vi "rt_loop_message_handling.vi"(8 "error in (no error)":errorcluster caption="错误输入（无错误）", 11 "Message Queues":T1 caption="消息队列") -> (0 "error out":errorcluster caption="错误输出")   [LabVIEW 2015]
uses:
  support_vis/message_queue/all_rt_message_queues.ctl
  support_vis/message_queue/message_cluster.ctl
  globals/global_monitoring_variables.vi
  globals/global_device_tree_items.vi
  globals/global_configuration_options.vi
  globals/global_all_rt_loop_stop.vi
  globals/global_rt_stream_connections.vi
  support_vis/message_queue/message_queue.lvlib
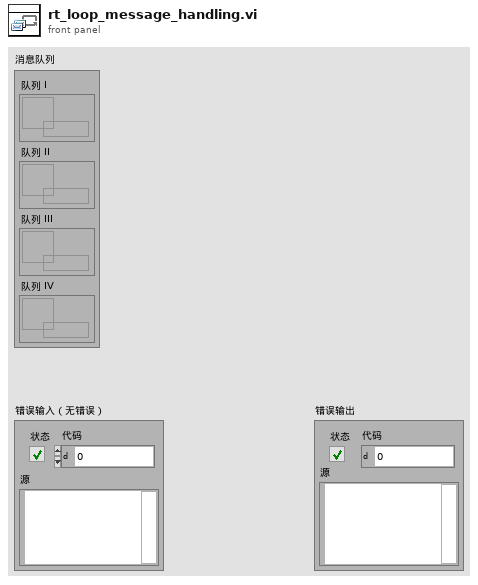
[diagram p1: front panel]
types:
  T1 = typedef "message_queue.lvlib/all_rt_message_queues.ctl" = cluster{"Queue I":refnum<queue>, "Queue II":refnum<queue>, "Queue III":refnum<queue>, "Queue IV":refnum<queue>}
  T2 = cluster{"Left Cell String":string, "Child Text":string[], "Child Tag":string, "Item Indent":i32, "Child Only?":bool, "Glyph Index":i32}[]
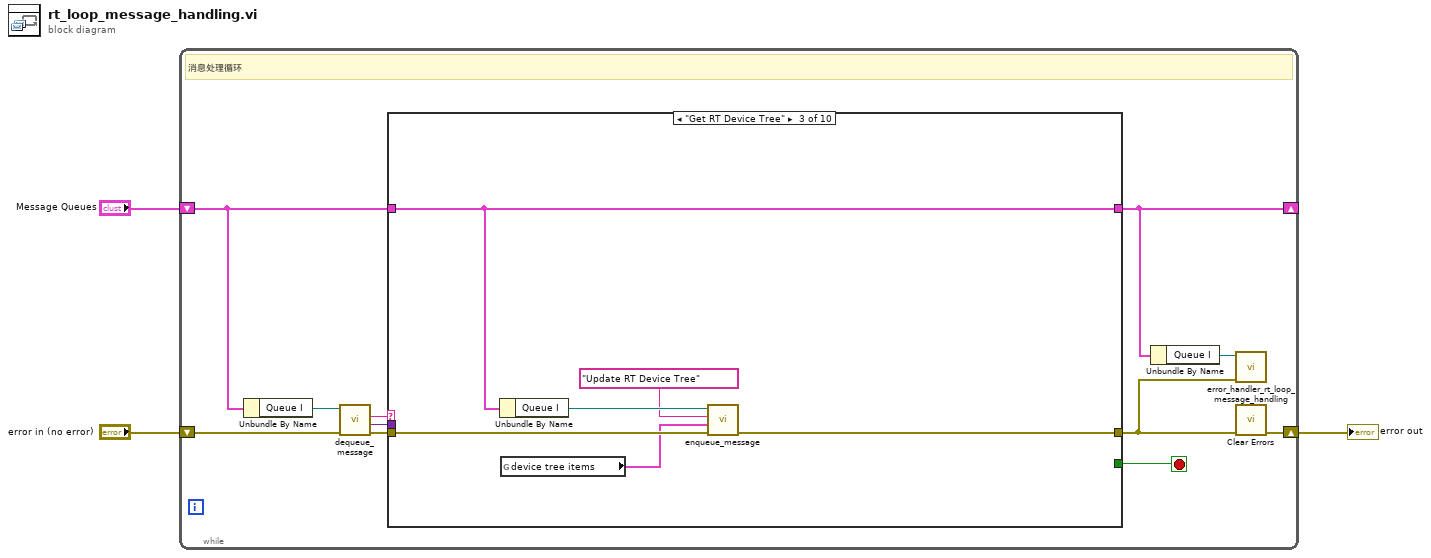
[diagram p0: block diagram]
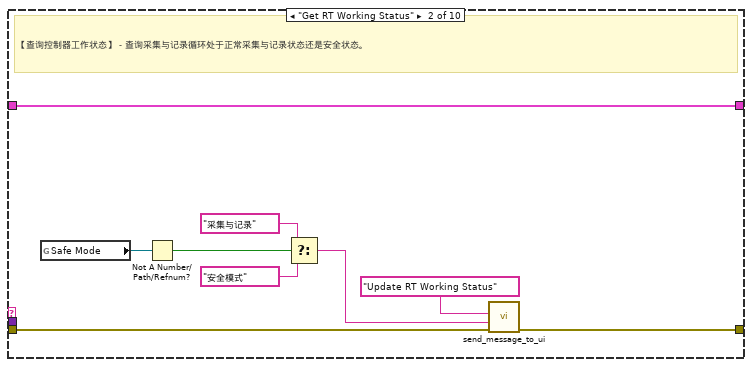
[diagram p3: hidden frame]
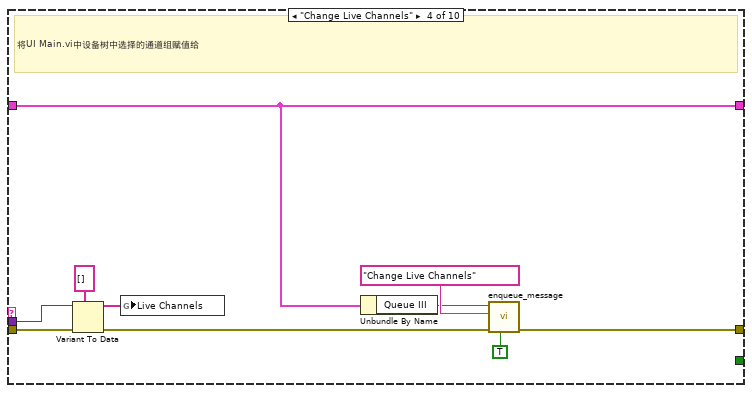
[diagram p4: hidden frame]
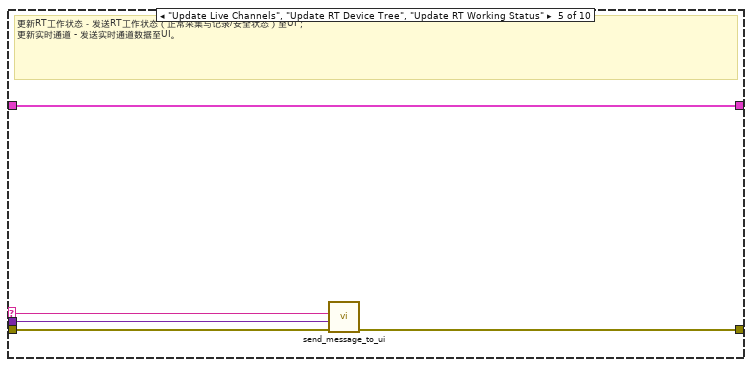
[diagram p5: hidden frame]
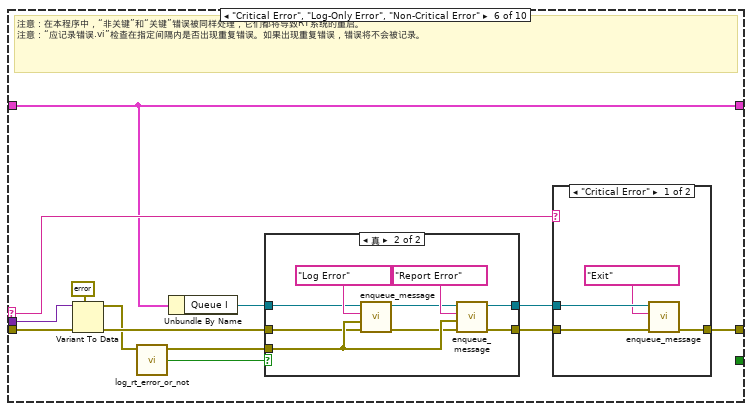
[diagram p6: hidden frame]
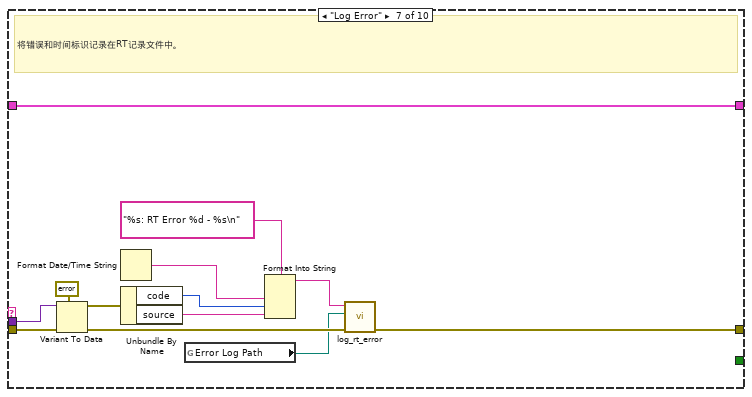
[diagram p9: hidden frame]
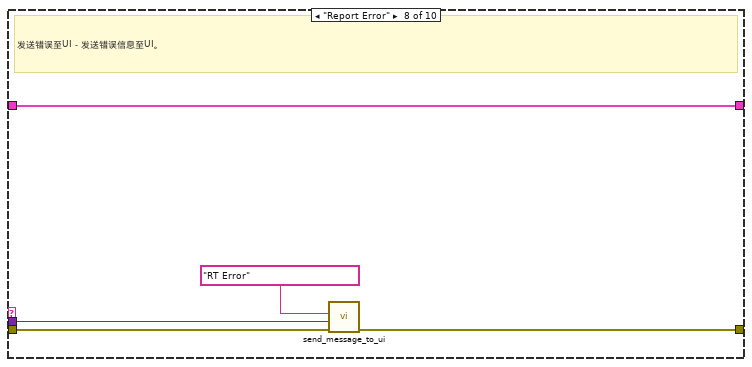
[diagram p10: hidden frame]
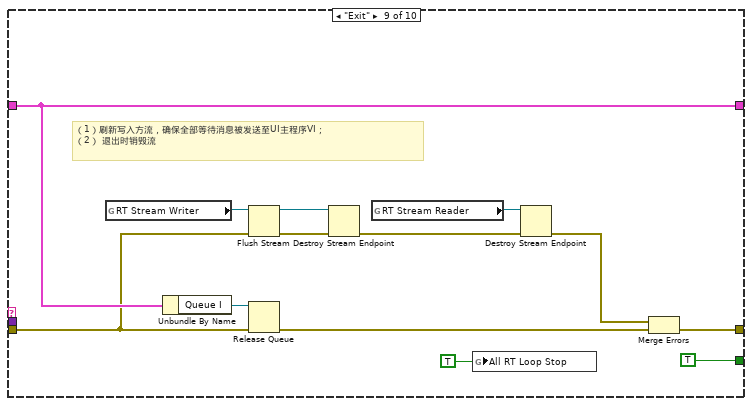
[diagram p11: hidden frame]
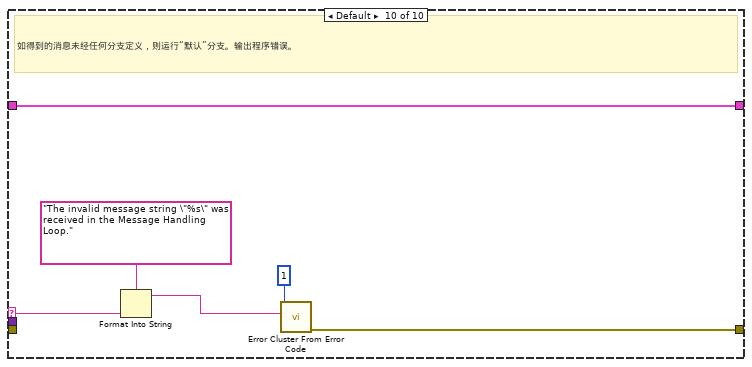
[diagram p12: hidden frame]
diagram:
  n1 = while {
    shift-right: [w9] -> w2
    shift-left: "error in (no error)" -> [w13]
    shift-right: [w6] -> _
    shift-left: "Message Queues" -> [w7]
    stop <- w14 stop-if-true
    # "消息处理循环"
    n2 = Unbundle By Name(w7) -> ("Queue I"=w5:refnum<queue>)
    n3 = call "dequeue_message.vi"("error in (no error)"=w13, "Message Queue"=w5) -> ("error out"=w12:errorcluster, "Message Data"=w10:variant, "Message"=w11:string)  [unwired: 6 in, 1 out]
    n4 = case "Message Cases" shown="\"Get RT Device Tree\"" w11 {
      selector: w11 -> [_ _ _ _ w42 w54 _ _ _ w111]
      tunnel: w12 -> [w16 w20 w27 w41 w46 w56 w88 w93 w96 _]
      tunnel: [w16 w19 w31 w36 w45 w59 w79 w92 w95 w109] -> w8
      tunnel: [_ _ _ _ _ _ _ _ TRUE _] -> w14
      tunnel: w10 -> [_ _ _ w39 w44 w49 w87 w91 _ _]
      tunnel: w7 -> [w15 w25 w30 w33 w43 w48 w76 w90 w99 w107]
      tunnel: [w15 w25 w30 w33 w43 w48 w76 w90 w99 w107] -> w6
      frame "Initialize" {
      }
      frame "Get RT Working Status" {
        # "【查询控制器工作状态】－查询采集与记录循环处于正常采集与记录状态还是安全状态。"
        n5 = global read "global_monitoring_variables.vi" "Safe Mode"() -> (w24:refnum<k4>)
        n6 = Not A Number/Path/Refnum?(number/path/refnum=w24) -> (NaN/Path/Refnum?=w23:bool)
        n7 = Select(t="采集与记录", s=w23, f="安全模式") -> (s? t:f=w18:string)
        n8 = call "send_message_to_ui.vi"("error in (no error)"=w20, "Message Data"=w18, "Message"="Update RT Working Status") -> ("error out"=w19:errorcluster)  [unwired: 8 in]
      }
      frame "Get RT Device Tree" {
        n9 = Unbundle By Name(w30) -> ("Queue I"=w29:refnum<queue>)
        n10 = global read "global_device_tree_items.vi" "device tree items"() -> (w26:T2)
        n11 = call "enqueue_message.vi"("error in (no error)"=w27, "Message Data"=w26, "Message"="Update RT Device Tree", "Message Queue"=w29) -> ("error out"=w31:errorcluster)  [unwired: 6 in, 1 out]
      }
      frame "Change Live Channels" {
        # "将UI Main.vi中设备树中选择的通道组赋值给"
        n12 = Variant To Data(error in=w41, type=string[] [] ("Displaying Channels"), Variant=w39) -> (data=w37:string[], error out=w40:errorcluster)
        n13 = global write "global_monitoring_variables.vi" "Live Channels"(w37) -> ()
        n14 = Unbundle By Name(w33) -> ("Queue III"=w32:refnum<queue>)
        n15 = call "enqueue_message.vi"("Priority Message? (F)"=TRUE, "error in (no error)"=w40, "Message"="Change Live Channels", "Message Queue"=w32) -> ("error out"=w36:errorcluster)  [unwired: 6 in, 1 out]
      }
      frame "Update Live Channels", "Update RT Device Tree", "Update RT Working Status" {
        # "更新RT工作状态－发送RT工作状态（正常采集与记录/安全状态）至UI；\n更新实时通道 - 发送实时通道数据至UI。"
        n16 = call "send_message_to_ui.vi"("error in (no error)"=w46, "Message Data"=w44, "Message"=w42) -> ("error out"=w45:errorcluster)  [unwired: 8 in]
      }
      frame "Critical Error", "Log-Only Error", "Non-Critical Error" {
        # "注意：在本程序中，“非关键”和“关键”错误被同样处理，它们都将导致RT系统的重启。\n注意：“应记录错误.vi”检查在指定间隔内是否出现重复错误。如果出现重复错误，错误将不会被记录。"
        n17 = Variant To Data(error in=w56, type=errorcluster {"status"=FALSE, "code"=0, "source"=""} ("error out"), Variant=w49) -> (data=w52:errorcluster, error out=w57:errorcluster)
        n18 = call "log_rt_error_or_not.vi"("error to report"=w52) -> ("Should Log Error?"=w50:bool, "dup error to report"=w51:errorcluster)  [unwired: 9 in]
        n19 = Unbundle By Name(w48) -> ("Queue I"=w47:refnum<queue>)
        n20 = case shown="真" w50 {
          tunnel: [w61 w68] -> w55
          tunnel: [w60 w67] -> w53
          tunnel: w47 -> [w60 w65]
          tunnel: w57 -> [w61 w62]
          tunnel: w51 -> [_ w66]
          frame False {
          }
          frame True {
            n21 = call "enqueue_message.vi"("error in (no error)"=w62, "Message Data"=w66, "Message"="Log Error", "Message Queue"=w65) -> ("error out"=w63:errorcluster, "dup Message Queue"=w64:refnum<queue>)  [unwired: 6 in]
            n22 = call "enqueue_message.vi"("error in (no error)"=w63, "Message Data"=w66, "Message"="Report Error", "Message Queue"=w64) -> ("error out"=w68:errorcluster, "dup Message Queue"=w67:refnum<queue>)  [unwired: 6 in]
          }
        }
        n23 = case shown="\"Critical Error\"" w54 {
          tunnel: w55 -> [w74 w75]
          tunnel: w53 -> [w72 _]
          tunnel: [w73 w75] -> w59
          frame "Critical Error" {
            n24 = call "enqueue_message.vi"("error in (no error)"=w74, "Message"="Exit", "Message Queue"=w72) -> ("error out"=w73:errorcluster)  [unwired: 7 in, 1 out]
          }
          frame Default {
          }
        }
      }
      frame "Log Error" {
        # "将错误和时间标识记录在RT记录文件中。"
        n25 = Variant To Data(error in=w88, type=errorcluster {"status"=FALSE, "code"=0, "source"=""} ("error constant"), Variant=w87) -> (data=w82:errorcluster, error out=w85:errorcluster)
        n26 = Format Date/Time String() -> (date/time string=w83:string)  [unwired: 3 in]
        n27 = Unbundle By Name(w82) -> ("code"=w81:i32, "source"=w80:string)
        n28 = global read "global_configuration_options.vi" "Error Log Path"() -> (w77:path)
        n29 = Format Into String(format string="%s: RT Error %d - %s\n", w83, w81, w80) -> (resulting string=w78:string)  [unwired: 2 in, 1 out]
        n30 = call "log_rt_error.vi"("error in (no error)"=w85, "Error Log Path"=w77, "Log Entry"=w78) -> ("error out"=w79:errorcluster)  [unwired: 8 in]
      }
      frame "Report Error" {
        # "发送错误至UI－发送错误信息至UI。"
        n31 = call "send_message_to_ui.vi"("error in (no error)"=w93, "Message Data"=w91, "Message"="RT Error") -> ("error out"=w92:errorcluster)  [unwired: 8 in]
      }
      frame "Exit" {
        # "（1）刷新写入方流，确保全部等待消息被发送至UI主程序VI；\n（2） 退出时销毁流"
        n32 = global read "global_rt_stream_connections.vi" "RT Stream Writer"() -> (w104:refnum<k21>)
        n33 = Unbundle By Name(w99) -> ("Queue I"=w98:refnum<queue>)
        n34 = Flush Stream(8:w96, 11:w104) -> (0:w100:errorcluster, 3:w101:refnum<k21>)  [unwired: 2 in, 1 out]
        n35 = Release Queue(queue=w98, error in (no error)=w96) -> (error out=w97:errorcluster)  [unwired: 1 in, 2 out]
        n36 = Destroy Stream Endpoint(8:w100, 11:w101) -> (0:w102:errorcluster)
        n37 = global read "global_rt_stream_connections.vi" "RT Stream Reader"() -> (w103:refnum<k21>)
        n38 = global write "global_all_rt_loop_stop.vi" "All RT Loop Stop"(TRUE ("Stop Monitoring Loops")) -> ()
        n39 = Destroy Stream Endpoint(8:w102, 11:w103) -> (0:w94:errorcluster)
        n40 = Merge Errors(w94, w97) -> (w95:errorcluster)
      }
      frame Default {
        # "如得到的消息未经任何分支定义，则运行“默认”分支。输出程序错误。"
        n41 = Format Into String(format string="The invalid message string \"%s\" was received in the Message Handling Loop." ("Unknown Message Error Text"), w111) -> (resulting string=w108:string)  [unwired: 2 in, 1 out]
        n42 = call <vilib>:"Error Cluster From Error Code.vi"("error message (\"\")"=w108, "error code (0)"=1) -> ("error out"=w109:errorcluster)  [unwired: 7 in]
      }
    }
    n43 = Unbundle By Name(w6) -> ("Queue I"=w4:refnum<queue>)
    n44 = call "error_handler_rt_loop_message_handling.vi"("error in (no error)"=w8, "Message Queue"=w4) -> ()  [unwired: 9 in, 1 out]
    n45 = call <vilib>:"Clear Errors.vi"("error in (no error)"=w8) -> ("error out"=w9:errorcluster)  [unwired: 5 in, 1 out]
  }
  "error out" <- w2
